vi "StartSequenceAcquisition.vi"(8 "error in (no error)":errorcluster, 10 "DataExchange":T1, 11 "Device in":refnum<class "Device.lvclass">) -> (0 "error out":errorcluster, 3 "Device out":refnum<class "Device.lvclass">)   [LabVIEW 2020, in "Device.lvlib" / "Device.lvclass"]
uses:
  Device.lvclass
  DataExchange.ctl
  DeviceStatus.ctl
  Device.lvclass/Device.ctl
  Device.lvlib
  Interface/DataListener/DataListener.lvclass
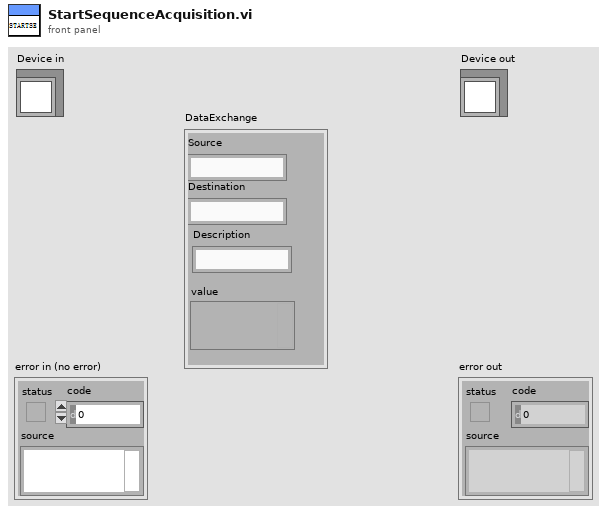
[diagram p1: front panel]
types:
  T1 = typedef "DataListener.lvclass/DataExchange.ctl" = cluster{"Source":string, "Destination":string, "Description":string, "value":variant}
  T2 = typedef "Device.lvlib/DeviceStatus.ctl" = i32
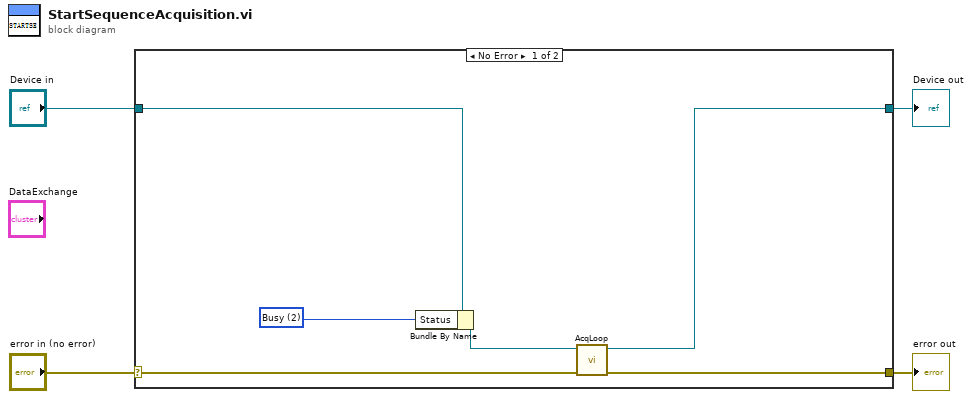
[diagram p0: block diagram]
diagram:
  n1 = case shown="No Error" "error in (no error)" {
    selector: "error in (no error)" -> [w10 w12]
    tunnel: [w9 w12] -> w3
    tunnel: [w8 w11] -> w1
    tunnel: "Device in" -> [w7 w11]
    frame No Error {
      w5 = T2 2 items=["Offline", "Idle", "Busy"] ("Status")
      n2 = Bundle By Name(cluster=w7, "Status"=w5) -> (w6:refnum<class "Device.lvclass">)
      n3 = call-dynamic "AcqLoop.vi"("error in (no error)"=w10, "Device in"=w6) -> ("error out"=w9:errorcluster, "Device out"=w8:refnum<class "Device.lvclass">)  [unwired: 8 in]
    }
    frame Error {
    }
  }
  "error out" <- w3
  "Device out" <- w1
